vi "UIM Reg Rtcn Call Back wrapper.vi"(8 "error in (no error)":errorcluster caption="错误输入（无错误）", 9 "user event":refnum<user-event>, 10 "dwDevIndex":u32, 11 "dwDevType":u16(ring)=4 items=["RS232CAN"=1, "WIFIRS232CAN"=2, "USBCAN"=4]) -> (0 "error out":errorcluster caption="错误输出", 3 "function return":u32)   [LabVIEW 2016, in "UISimCanFunc_wrapper.lvlib"]
doc: "_declspec (dllexport) DWORD UIMRegRtcnCallBack_wrapper(DWORD dwDevType, DWORD dwDevIndex, LVUserEventRef *rwer);"
uses:
  <userlib>/UISimCanFunc_wrapper/UISimCanFunc_wrapper.lvlib
  <userlib>/UISimCanFunc_wrapper/UISimCanFunc_wrapper.dll
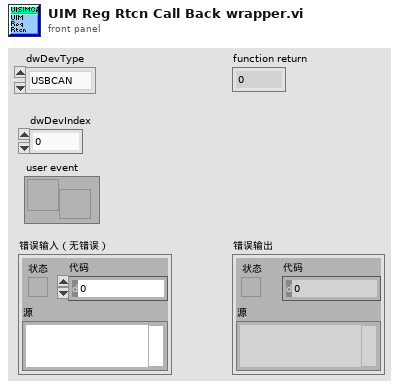
[diagram p1: front panel]
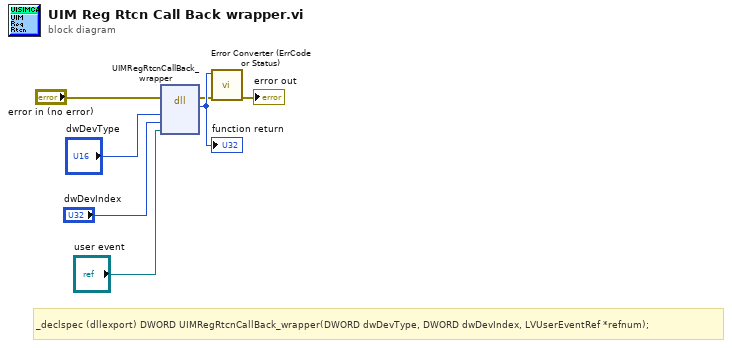
[diagram p0: block diagram]
diagram:
  # "_declspec (dllexport) DWORD UIMRegRtcnCallBack_wrapper(DWORD dwDevType, DWORD dwDevIndex, LVUserEventRef *refnum);"
  n1 = dll-call lib="C:/Program Files (x86)/National Instruments/LabVIEW 2016/user.lib/UISimCanFunc_wrapper/UISimCanFunc_wrapper.*" fn="UIMRegRtcnCallBack_wrapper"(error in="error in (no error)", "dwDevType"="dwDevType", "dwDevIndex"="dwDevIndex", "refnum"="user event") -> (error out=w4:errorcluster, "返回类型"=w7:u32)  [unwired: 5 in, 1 out]
  "function return" <- w7
  n2 = call <userlib>:"Error Converter (ErrCode or Status).vi"("error in (no error)"=w4, "error code"=w7) -> ("error out"=→"error out":errorcluster)  [unwired: 9 in]
